vi "water flow controller.vi"(4 "State":i16, 5 "Time":dbl format="%.2f", 6 "Sensor Values":dbl[](array[numeric]), 7 "Set Points":dbl[](array[numeric])) -> (0 "required data":T1={"Set Point names"=["flow rate (mL/min", "P Kc", "I Ti (min)", "D Td (min)"], "required number of setpoints"=4, "required number of sensors"=1, "Sensor names"=["flow sensor"]}, 3 "output value":dbl)   [LabVIEW 2019]
uses:
  PID library.llb/PID (DBL).vi
panel:
  # "Enter the correct information for this control code in the required data structure below. Then make the current value default by right clicking on the border of the data structure."
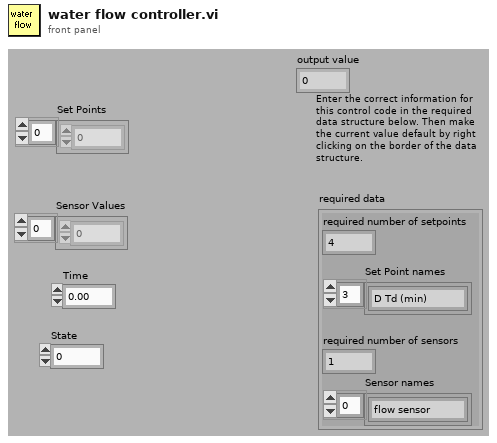
[diagram p1: front panel]
types:
  T1 = cluster{"Set Point names":string[], "required number of setpoints":u8, "required number of sensors":u8, "Sensor names":string[]}
  T2 = cluster{"Sensor Values[0]":dbl, "Sensor Values[1]":dbl, "Sensor Values[2]":dbl, "Sensor Values[3]":dbl}
  T3 = cluster{"Sensor Values[1]":dbl, "Sensor Values[2]":dbl, "Sensor Values[3]":dbl}
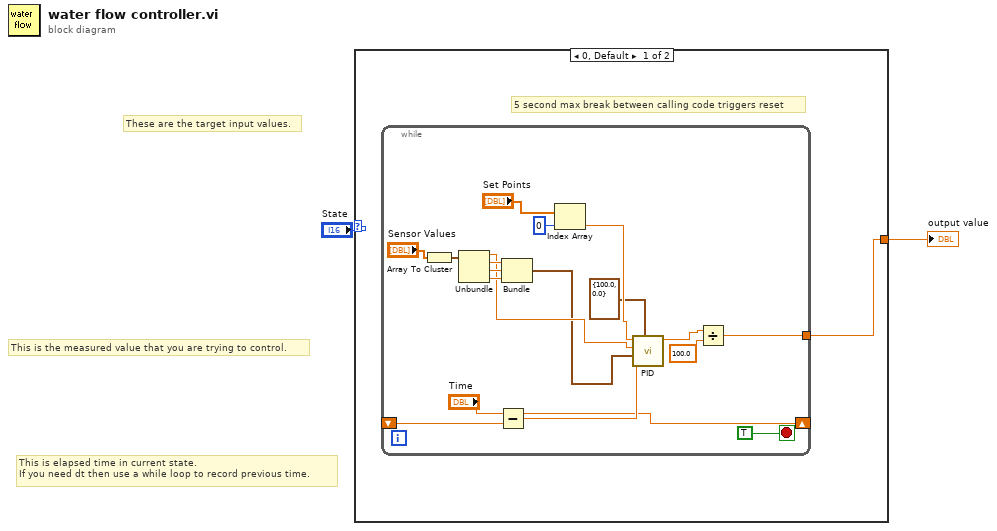
[diagram p0: block diagram]
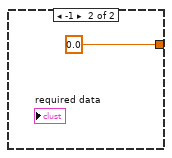
[diagram p2: hidden frame]
diagram:
  # "These are the target input values."
  # "This is the measured value that you are trying to control."
  # "This is elapsed time in current state.\nIf you need dt then use a while loop to record previous time."
  n1 = case shown="0, Default" "State" {
    tunnel: [w3 0.0 ("fraction on")] -> w1
    frame 0, Default {
      # "5 second max break between calling code triggers reset"
      n2 = while {
        shift-right: ["Time"] -> _
        shift-left: _ -> [w19]
        tunnel: [w11] -> w3
        stop <- TRUE stop-if-true
        n3 = Array To Cluster(array="Sensor Values") -> (cluster=w10:T2)
        n4 = Unbundle(w10) -> ("Sensor Values[0]"=w5:dbl, "Sensor Values[1]"=w8:dbl, "Sensor Values[2]"=w9:dbl, "Sensor Values[3]"=w7:dbl)
        n5 = Subtract(x="Time", y=w19) -> (x-y=w18:dbl)
        n6 = Bundle("Sensor Values[1]"=w8, "Sensor Values[2]"=w9, "Sensor Values[3]"=w7) -> (w4:T3)  [unwired: 1 in]
        n7 = Index Array(array="Set Points", index=0) -> (element=w20:dbl)
        n8 = call-poly "PID.vi"("output range"=cluster{"output high":dbl, "output low":dbl} {"output high"=100.0, "output low"=0.0}, "dt (s)"=w18, "PID gains"=w4, "process variable"=w5, "setpoint"=w20) -> ("output"=w16:dbl)  [unwired: 5 in, 1 out]
        n9 = Divide(x=w16, y=100.0) -> (x/y=w11:dbl)
      }
    }
    frame -1 {
    }
  }
  "output value" <- w1
